vi "atcs_monitorCommand_SpectrographSetup.vi"(8 "error in (no error)":errorcluster, 11 "command_SpectrographSetup_Ctl":T1) -> (0 "error out":errorcluster, 2 "function return":i32, 3 "command_SpectrographSetup_Ctl out":T1)   [LabVIEW 2016, in "SALLV_atcs.lvlib"]
doc: "int atcs_shm_monitorCommand_SpectrographSetupLV(atcs_command_SpectrographSetupLV *command_SpectrographSetup_Ctl );"
uses:
  SALLV_atcs.lvlib
  DataTypes/command_SpectrographSetup.ctl
  SALLV_atcs.so
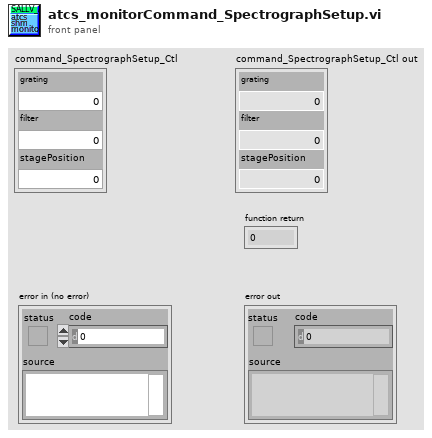
[diagram p1: front panel]
types:
  T1 = typedef "SALLV_atcs.lvlib/command_SpectrographSetup.ctl" = cluster{"grating":i32, "filter":i32, "stagePosition":dbl}
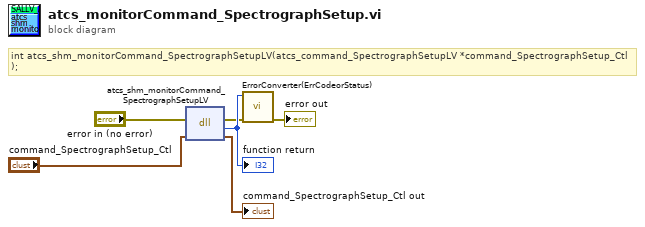
[diagram p0: block diagram]
diagram:
  # "int atcs_shm_monitorCommand_SpectrographSetupLV(atcs_command_SpectrographSetupLV *command_SpectrographSetup_Ctl );"
  n1 = dll-call lib="home/andres/Desktop/SALLV_atcs/SALLV_atcs.*" fn="atcs_shm_monitorCommand_SpectrographSetupLV"(error in="error in (no error)", "command_SpectrographSetup_Ctl"="command_SpectrographSetup_Ctl") -> (error out=w2:errorcluster, w6:i32, "command_SpectrographSetup_Ctl"=→"command_SpectrographSetup_Ctl out":T1)  [unwired: 2 in, 1 out]
  "function return" <- w6
  n2 = call "ErrorConverter(ErrCodeorStatus).vi"("error in (no error)"=w2, "error code"=w6) -> ("error out"=→"error out":errorcluster)  [unwired: 9 in]
